vi "End.vi"(8 "error in (no error)":errorcluster, 11 "Channel GUI in":refnum<class "Channel GUI.lvclass">) -> (0 "error out":errorcluster, 3 "Channel GUI out":refnum<class "Channel GUI.lvclass">)   [LabVIEW 2018, in "Channel GUI.lvclass"]
uses:
  Channel GUI.lvclass
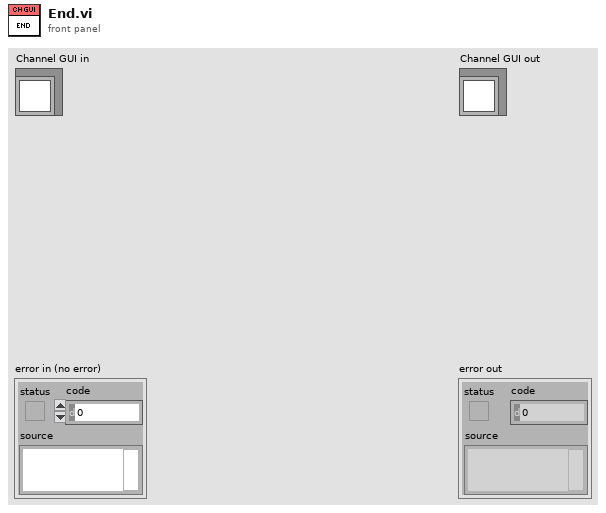
[diagram p1: front panel]
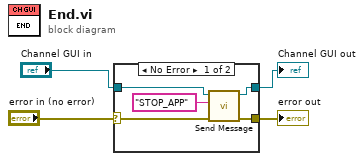
[diagram p0: block diagram]
diagram:
  n1 = case shown="No Error" "error in (no error)" {
    selector: "error in (no error)" -> [w6 w11]
    tunnel: [w8 w11] -> w2
    tunnel: [w5 w10] -> w1
    tunnel: "Channel GUI in" -> [w7 w10]
    frame No Error {
      n2 = call "Send Message.vi"("error in (no error)"=w6, "Message"="STOP_APP", "Channel GUI in"=w7) -> ("error out"=w8:errorcluster, "Channel GUI out"=w5:refnum<class "Channel GUI.lvclass">)  [unwired: 7 in]
    }
    frame Error {
    }
  }
  "error out" <- w2
  "Channel GUI out" <- w1
